vi "Clear_Info.vi"(8 "error in (no error)":errorcluster, 9 "index":string, 10 "buildObject":T1, 11 "IB_Destination.lvclass":refnum<class "IB_Destination.lvclass">) -> (0 "error out":errorcluster, 3 "IB_Destination out":refnum<class "IB_Destination.lvclass">)   [LabVIEW 2020, in "IB_Destination.lvclass"]
uses:
  <vilib>/AppBuilder/IB_Classes/Destination/IB_Destination.lvclass
  <vilib>/AppBuilder/IB_Classes/Destination/IB_Destination.lvclass/IB_Destination.ctl
  <vilib>/AppBuilder/IB_RW_Project/IB_RW_Project_PropBag_Action.ctl
  <resource>/Framework/Providers/API/ItemRef.ctl
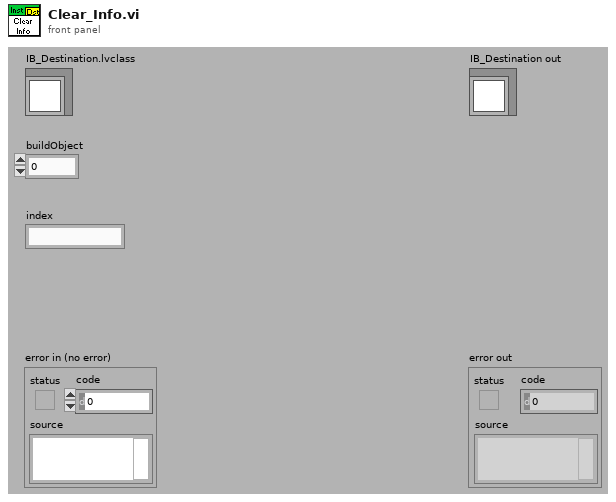
[diagram p1: front panel]
types:
  T1 = typedef "ItemRef.ctl" = u64
  T2 = typedef "IB_RW_Project_PropBag_Action.ctl" = enum16{"read", "write", "clear", "readPrevious", "writePrevious", "clearPrevious"}
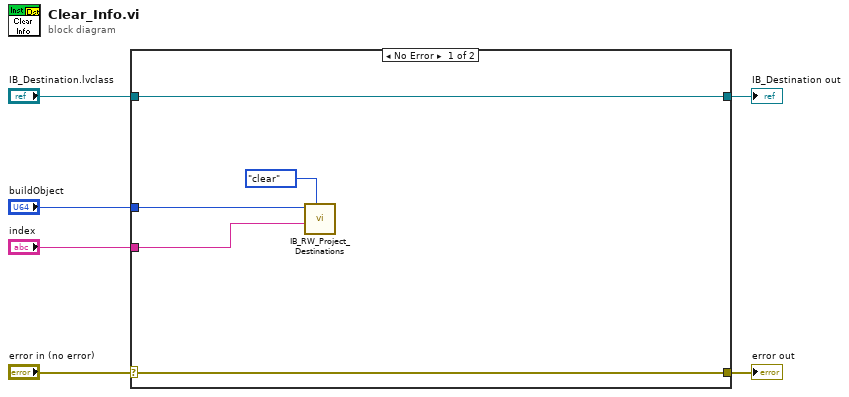
[diagram p0: block diagram]
diagram:
  n1 = case shown="No Error" "error in (no error)" {
    selector: "error in (no error)" -> [w11 w13]
    tunnel: [w11 w13] -> w5
    tunnel: [w7 w12] -> w3
    tunnel: "IB_Destination.lvclass" -> [w7 w12]
    tunnel: "buildObject" -> [w9 _]
    tunnel: "index" -> [w8 _]
    frame No Error {
      n2 = call <vilib>:"IB_RW_Project_Destinations.vi"("action"=IB_RW_Project_PropBag_Action."clear", "index"=w8, "buildObject"=w9) -> ()  [unwired: 5 in, 4 out]
    }
    frame Error {
    }
  }
  "error out" <- w5
  "IB_Destination out" <- w3
